vi "Get State.vi"(8 "error in (no error)":errorcluster, 11 "System Actor in":refnum<class "System Actor.lvclass">) -> (0 "error out":errorcluster, 1 "System State String":string, 3 "System Actor out":refnum<class "System Actor.lvclass">)   [LabVIEW 2014, in "Robot Actor Framework.lvlib" / "System Actor.lvlib" / "System Actor.lvclass"]
uses:
  System Actor.lvclass
  System Actor.lvclass/System Actor.ctl
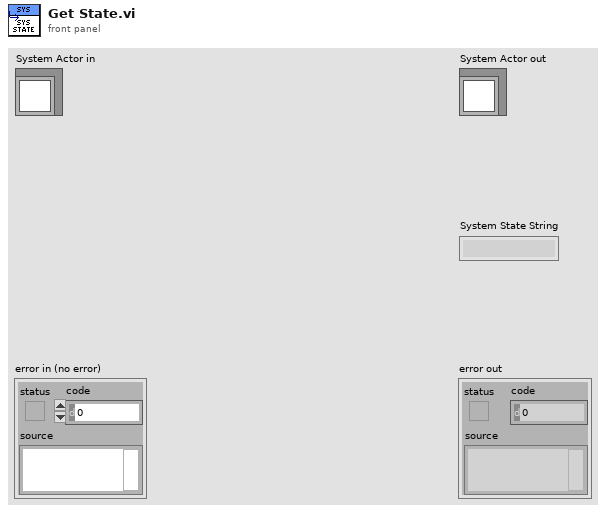
[diagram p1: front panel]
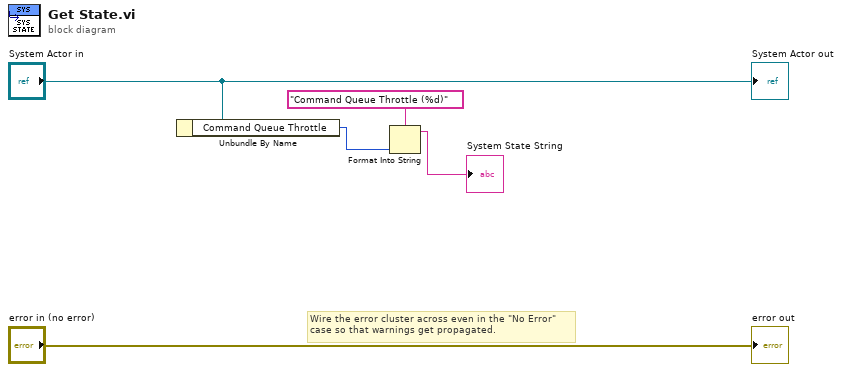
[diagram p0: block diagram]
diagram:
  # "Wire the error cluster across even in the \"No Error\"\ncase so that warnings get propagated."
  n1 = Unbundle By Name("System Actor in") -> ("Command Queue Throttle"=w2:u32)
  n2 = Format Into String(format string="Command Queue Throttle (%d)", w2) -> (resulting string=→"System State String":string)  [unwired: 2 in, 1 out]
  "error out" <- "error in (no error)"
  "System Actor out" <- "System Actor in"
